vi "Begin.vi"(11 "Image Size":T1=enum."320x240") -> (0 "error out":errorcluster)   [LabVIEW 2012]
doc: "Called before other user functions, this VI is expected to open initial I/O refnums, load in file data, and do all program initialization. Notice that the <B>error out</B> terminal is simply used for data flow. Wiring it to other structures or subVIs ensures that this VI runs first."
uses:
  <vilib>/Rock Robotics/WPI/Camera/WPI_CameraImageSize.ctl
  <vilib>/Rock Robotics/WPI/DriverStation/WPI_DriverStationRobotMode2.ctl
  <vilib>/Rock Robotics/SystemInterfaces/DIO/FPGA_DIOPWMChannel.ctl
  <vilib>/Rock Robotics/WPI/Joystick/WPI_JoystickDeviceEnum.ctl
  <vilib>/Rock Robotics/SystemInterfaces/Typedef/FPGA_TypedefDigitalModule.ctl
  <vilib>/Rock Robotics/WPI/Relay/WPI_RelayDirection.ctl
  <vilib>/Rock Robotics/SystemInterfaces/DIO/FPGA_DIORelayChannel.ctl
  <vilib>/Rock Robotics/SystemInterfaces/AI/FPGA_AIChannel.ctl
  <vilib>/Rock Robotics/SystemInterfaces/AI/FPGA_AIGyroChannel.ctl
  <vilib>/Rock Robotics/SystemInterfaces/DIO/FPGA_DIOChannel.ctl
  <vilib>/Rock Robotics/WPI/Camera/WPI_CameraFrameRate.ctl
  Robot Global Data.vi
  <vilib>/Rock Robotics/WPI/MotorControl/WPI_MotorControlOpen Victor.vi
  <vilib>/Rock Robotics/WPI/Camera/WPI_CameraWhite Balance Values.ctl
  <vilib>/Rock Robotics/WPI/Camera/WPI_CameraExposure Values.ctl
  <vilib>/Rock Robotics/WPI/MotorControl/WPI_MotorControlOpen Jaguar.vi
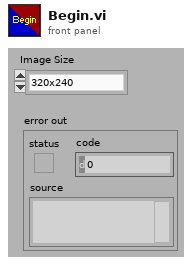
[diagram p1: front panel]
types:
  T1 = typedef "WPI_CameraImageSize.ctl" = enum16{"640x480", "320x240", "160x120"}
  T2 = typedef "FPGA_AIChannel.ctl" = enum8{"AI 1", "AI 2", "AI 3", "AI 4", "AI 5", "AI 6", "AI 7", "AI 8", "Invalid"}
  T3 = typedef "FPGA_DIOChannel.ctl" = enum8{"DIO 1", "DIO 2", "DIO 3", "DIO 4", "DIO 5", "DIO 6", "DIO 7", "DIO 8", "DIO 9", "DIO 10", "DIO 11", "DIO 12", "DIO 13", "DIO 14", "Invalid"}
  T4 = typedef "FPGA_TypedefDigitalModule.ctl" = enum16{"Digital Module 1", "Digital Module 2"}
  T5 = typedef "FPGA_DIOPWMChannel.ctl" = enum8{"PWM 1", "PWM 2", "PWM 3", "PWM 4", "PWM 5", "PWM 6", "PWM 7", "PWM 8", "PWM 9", "PWM 10", "Invalid"}
  T6 = typedef "FPGA_AIGyroChannel.ctl" = enum8{"AI 1", "AI 2", "Invalid"}
  T7 = typedef "FPGA_DIORelayChannel.ctl" = enum8{"Relay 1", "Relay 2", "Relay 3", "Relay 4", "Relay 5", "Relay 6", "Relay 7", "Relay 8", "Invalid"}
  T8 = typedef "WPI_RelayDirection.ctl" = enum16{"Both directions", "Forward only", "Reverse only"}
  T9 = typedef "WPI_JoystickDeviceEnum.ctl" = enum16{"USB 1", "USB 2", "USB 3", "USB 4", "Kinect 1", "Kinect 2"}
  T10 = typedef "WPI_DriverStationRobotMode2.ctl" = enum16{"Autonomous Disabled", "Autonomous Enabled", "Teleop Disabled", "Teleop Enabled", "Timeout", "Finish", "Test Disabled", "Test Enabled"}
  T11 = typedef "WPI_CameraFrameRate.ctl" = u32
  T12 = typedef "WPI_CameraExposure Values.ctl" = enum16{"Auto", "Flicker-free 50 Hz", "Flicker-free 60 Hz", "Hold current"}
  T13 = typedef "WPI_CameraWhite Balance Values.ctl" = enum16{"Auto", "Fixed indoor", "Fixed outdoor 1", "Fixed outdoor 2", "Fixed fluorescent 1", "Fixed fluorescent 2", "Hold current"}
  T14 = typedef "WPI_CameraDevRef.ctl" = cluster{"Camera Address":string, "CameraStatus":errorcluster, "Acquire Image Notifier":refnum<notifier>}
  T15 = typedef "WPI_MotorControlDeviceRef.ctl" = cluster{"DeviceStatus":errorcluster, "Type":enum16{"PWM", "CAN"}, "PWM":cluster{"Digital Module":T4, "PWM Channel":T5, "DeadBand":T16}, "CAN":cluster{"Device Number":u8, "Control Mode":T17, "Semaphore":T18, "Max Vout":dbl}, "Invert":bool, "TransformRef":T19, "InvTransformRef":T19}
  T16 = typedef "WPI_PWMDeadband.ctl" = cluster{"Name":string, "maxPositivePwm":i32, "minPositivePwm":i32, "centerPwm":i32, "maxNegativePwm":i32, "minNegativePwm":i32, "angularRange":u16}
  T17 = typedef "WPI_CANJaguar_ControlMode.ctl" = enum8{"Percent VBus", "Current", "Speed", "Position", "Voltage"}
  T18 = typedef "Semaphore RefNum" = refnum<k1>
  T19 = typedef "WPI_PWMTransform_ConPane.ctl" = refnum<vi>
  T20 = typedef "WPI_JoystickDevRef.ctl" = cluster{"Device":T9}
  T21 = typedef "WPI_ServoDeviceRef.ctl" = cluster{"DeviceStatus":errorcluster, "Digital Module":T4, "PWM Channel":T5, "DeadBand":T16}
  T22 = typedef "WPI_RelayDevRef.ctl" = cluster{"DevStatus":errorcluster, "Relay Channel":T7, "Digital Module":T4, "Relay Direction":T8}
  T23 = typedef "WPI_AnalogChannelDevRef.ctl" = cluster{"DevStatus":errorcluster, "Analog Module":T24, "Analog Channel":T2}
  T24 = typedef "FPGA_TypedefAnalogModule.ctl" = enum16{"Analog Module 1", "Analog Module 2"}
  T25 = typedef "WPI_DigitalInputDevRef.ctl" = cluster{"DevStatus":errorcluster, "DIO Channel":T3, "Digital Module":T4}
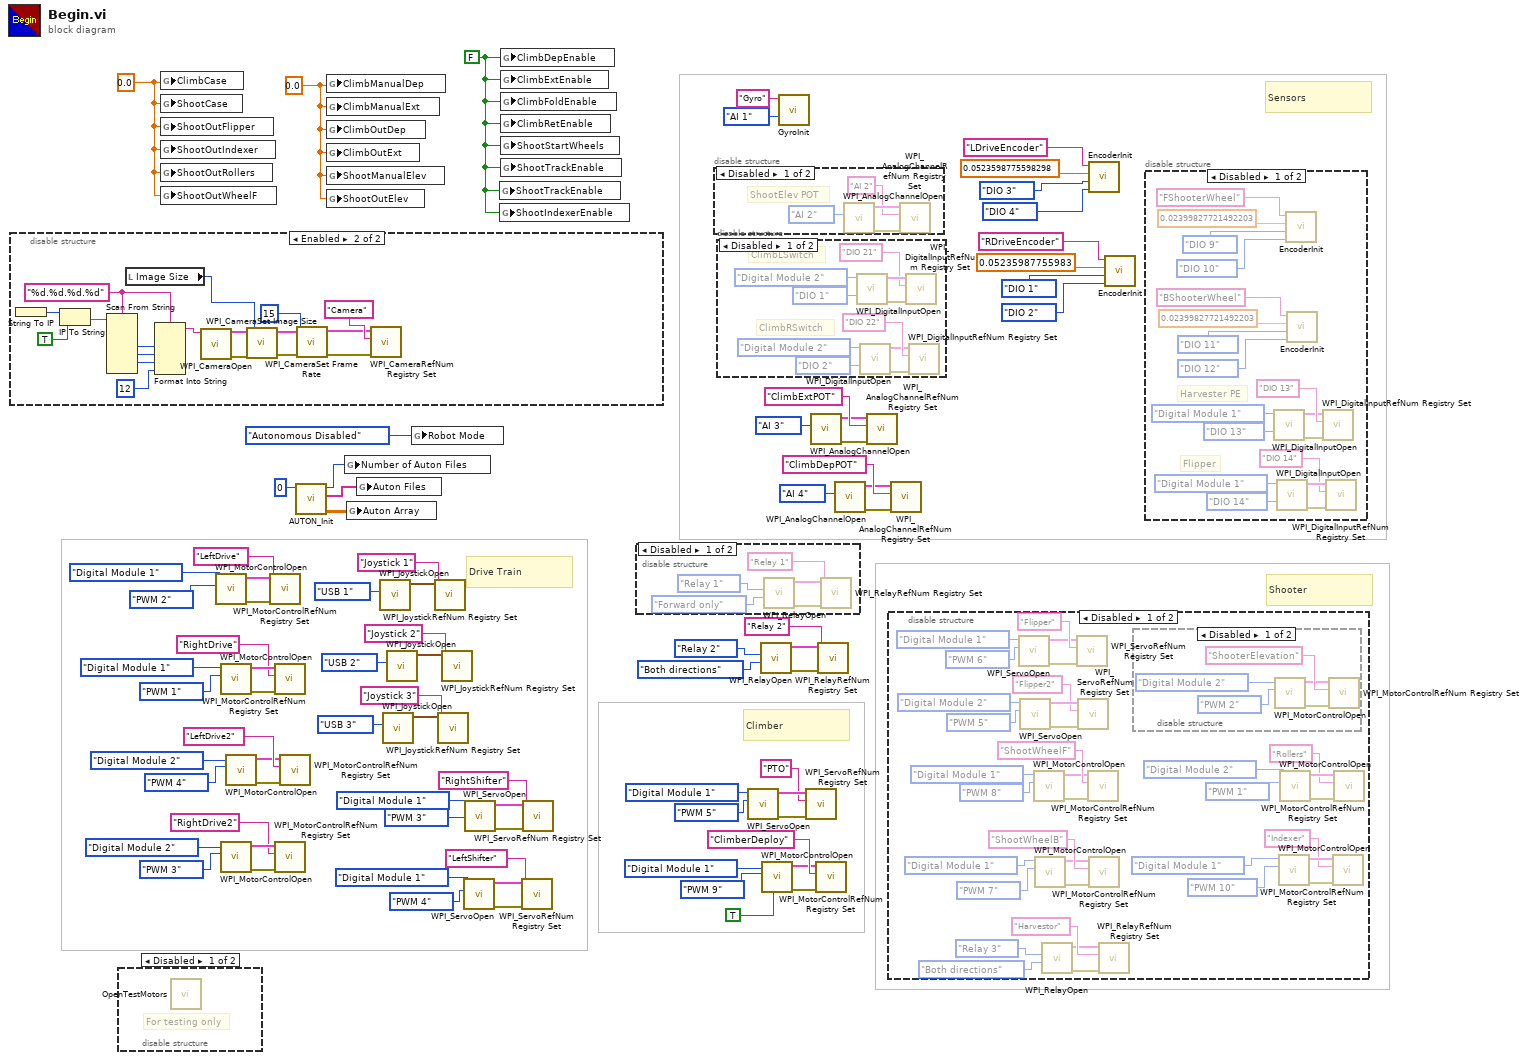
[diagram p0: block diagram]
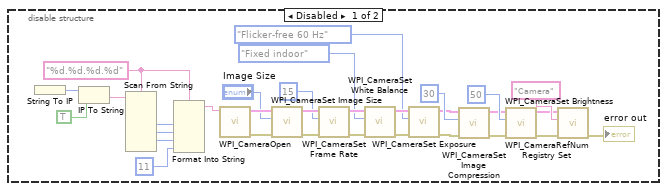
[diagram p6: hidden frame]
diagram:
  w57 = FALSE ("ClimbDepEnable")
  w58 = 0.0 ("ClimbCase")
  w59 = 0.0 ("ClimbCase")
  # "Drive Train"
  # "Climber"
  # "Shooter"
  # "Sensors"
  n1 = disable-structure shown="Enabled" {
    frame Disabled {
      w84 = "%d.%d.%d.%d" ("format string")
      n2 = String To IP() -> (0:w91:u32)  [unwired: 1 in]
      n3 = IP To String(1:TRUE ("dot notation? (F)"), 2:w91) -> (0:w89:string)
      n4 = Scan From String(format string=w84, input string=w89) -> (output 1=w88:i32, output 2=w87:i32, output 3=w86:i32)  [unwired: 7 in, 3 out]
      n5 = Format Into String(format string=w84, w88, w87, w86, 11 ("Compression")) -> (resulting string=w83:string)  [unwired: 2 in, 1 out]
      n6 = call <vilib>:"WPI_CameraOpen.vi"("Camera Address"=w83) -> ("error out"=w103:errorcluster, "CameraDevRef"=w104:T14)  [unwired: 1 in, 8 out]
      n7 = call <vilib>:"WPI_CameraSet Image Size.vi"("error in (no error)"=w103, "Image Size"="Image Size", "CameraDevRef"=w104) -> ("error out"=w102:errorcluster, "CameraDevRef Out"=w105:T14)  [unwired: 7 out]
      n8 = call <vilib>:"WPI_CameraSet Frame Rate.vi"("error in (no error)"=w102, "Frame Rate (fps)"=T11 15, "CameraDevRef"=w105) -> ("error out"=w101:errorcluster, "CameraDevRef Out"=w107:T14)  [unwired: 7 out]
      n9 = call <vilib>:"WPI_CameraSet White Balance.vi"("error in (no error)"=w101, "White Balance"=WPI_CameraWhite_Balance_Values."Fixed indoor", "CameraDevRef"=w107) -> ("error out"=w100:errorcluster, "CameraDevRef Out"=w106:T14)  [unwired: 7 out]
      n10 = call <vilib>:"WPI_CameraSet Exposure.vi"("error in (no error)"=w100, "Exposure"=WPI_CameraExposure_Values."Flicker-free 60 Hz", "CameraDevRef"=w106) -> ("error out"=w99:errorcluster, "CameraDevRef Out"=w109:T14)  [unwired: 7 out]
      n11 = call <vilib>:"WPI_CameraSet Image Compression.vi"("error in (no error)"=w99, "Compression"=30, "CameraDevRef"=w109) -> ("error out"=w98:errorcluster, "CameraDevRef Out"=w108:T14)  [unwired: 7 out]
      n12 = call <vilib>:"WPI_CameraSet Brightness.vi"("error in (no error)"=w98, "Brightness"=50, "CameraDevRef"=w108) -> ("error out"=w96:errorcluster, "CameraDevRef Out"=w97:T14)  [unwired: 7 out]
      n13 = call <vilib>:"WPI_CameraRefNum Registry Set.vi"("error in (no error)"=w96, "refnum name"="Camera", "CameraDevRef"=w97) -> ("error out"=→"error out":errorcluster)  [unwired: 8 out]
    }
    frame Enabled {
      w122 = "%d.%d.%d.%d" ("format string")
      n14 = String To IP() -> (0:w129:u32)  [unwired: 1 in]
      n15 = IP To String(1:TRUE ("dot notation? (F)"), 2:w129) -> (0:w127:string)
      n16 = Scan From String(format string=w122, input string=w127) -> (output 1=w126:i32, output 2=w125:i32, output 3=w124:i32)  [unwired: 7 in, 3 out]
      n17 = local read "Image Size"() -> (w118:T1)
      n18 = Format Into String(format string=w122, w126, w125, w124, 12 ("Compression")) -> (resulting string=w121:string)  [unwired: 2 in, 1 out]
      n19 = call <vilib>:"WPI_CameraOpen.vi"("Camera Address"=w121) -> ("error out"=w120:errorcluster, "CameraDevRef"=w119:T14)  [unwired: 1 in, 8 out]
      n20 = call <vilib>:"WPI_CameraSet Image Size.vi"("error in (no error)"=w120, "Image Size"=w118, "CameraDevRef"=w119) -> ("error out"=w116:errorcluster, "CameraDevRef Out"=w117:T14)  [unwired: 7 out]
      n21 = call <vilib>:"WPI_CameraSet Frame Rate.vi"("error in (no error)"=w116, "Frame Rate (fps)"=T11 15, "CameraDevRef"=w117) -> ("error out"=w115:errorcluster, "CameraDevRef Out"=w114:T14)  [unwired: 7 out]
      n22 = call <vilib>:"WPI_CameraRefNum Registry Set.vi"("error in (no error)"=w115, "refnum name"="Camera", "CameraDevRef"=w114) -> ()  [unwired: 9 out]
    }
  }
  n23 = disable-structure shown="Disabled" {
    frame Disabled {
      # "For testing only"
      n24 = call "OpenTestMotors.vi"() -> ()  [unwired: 12 in]
    }
    frame Enabled {
    }
  }
  n25 = global write "Robot Global Data.vi" "ClimbCase"(w59) -> ()
  n26 = global write "Robot Global Data.vi" "ShootCase"(w59) -> ()
  n27 = global write "Robot Global Data.vi" "ShootOutFlipper"(w59) -> ()
  n28 = global write "Robot Global Data.vi" "ShootOutIndexer"(w59) -> ()
  n29 = global write "Robot Global Data.vi" "ShootOutRollers"(w59) -> ()
  n30 = global write "Robot Global Data.vi" "ShootOutWheelF"(w59) -> ()
  n31 = call-poly <vilib>:"WPI_MotorControlOpen.vi"("PWM Channel"=FPGA_DIOPWMChannel."PWM 2", "Digital Module (Module 1)"=FPGA_TypedefDigitalModule."Digital Module 1") -> ("error out"=w69:errorcluster, "MotorControlDeviceRef"=w70:T15)  [unwired: 8 in]
  n32 = call-poly <vilib>:"WPI_MotorControlOpen.vi"("PWM Channel"=FPGA_DIOPWMChannel."PWM 1", "Digital Module (Module 1)"=FPGA_TypedefDigitalModule."Digital Module 1") -> ("error out"=w76:errorcluster, "MotorControlDeviceRef"=w75:T15)  [unwired: 8 in]
  n33 = call-poly <vilib>:"WPI_MotorControlOpen.vi"("PWM Channel"=FPGA_DIOPWMChannel."PWM 3", "Digital Module (Module 1)"=FPGA_TypedefDigitalModule."Digital Module 2") -> ("error out"=w55:errorcluster, "MotorControlDeviceRef"=w54:T15)  [unwired: 8 in]
  n34 = call-poly <vilib>:"WPI_MotorControlOpen.vi"("PWM Channel"=FPGA_DIOPWMChannel."PWM 4", "Digital Module (Module 1)"=FPGA_TypedefDigitalModule."Digital Module 2") -> ("error out"=w46:errorcluster, "MotorControlDeviceRef"=w47:T15)  [unwired: 8 in]
  n35 = call <vilib>:"WPI_MotorControlRefNum Registry Set.vi"("error in (no error)"=w69, "refnum name"="LeftDrive", "MotorControlDevRef"=w70) -> ()  [unwired: 7 in, 2 out]
  n36 = call <vilib>:"WPI_MotorControlRefNum Registry Set.vi"("error in (no error)"=w76, "refnum name"="RightDrive", "MotorControlDevRef"=w75) -> ()  [unwired: 7 in, 2 out]
  n37 = call <vilib>:"WPI_MotorControlRefNum Registry Set.vi"("error in (no error)"=w55, "refnum name"="RightDrive2", "MotorControlDevRef"=w54) -> ()  [unwired: 7 in, 2 out]
  n38 = call <vilib>:"WPI_MotorControlRefNum Registry Set.vi"("error in (no error)"=w46, "refnum name"="LeftDrive2", "MotorControlDevRef"=w47) -> ()  [unwired: 7 in, 2 out]
  n39 = call "AUTON_Init.vi"("Default File"=0) -> ("Auton Array"=w77:dbl[][], "Auton Files"=w78:string[], "Number of Auton Files"=w79:i64)  [unwired: 8 in]
  n40 = global write "Robot Global Data.vi" "ClimbManualDep"(w58) -> ()
  n41 = global write "Robot Global Data.vi" "ClimbManualExt"(w58) -> ()
  n42 = global write "Robot Global Data.vi" "ClimbOutDep"(w58) -> ()
  n43 = global write "Robot Global Data.vi" "ClimbOutExt"(w58) -> ()
  n44 = global write "Robot Global Data.vi" "ShootManualElev"(w58) -> ()
  n45 = global write "Robot Global Data.vi" "ShootOutElev"(w58) -> ()
  n46 = global write "Robot Global Data.vi" "Number of Auton Files"(w79) -> ()
  n47 = global write "Robot Global Data.vi" "Auton Array"(w77) -> ()
  n48 = global write "Robot Global Data.vi" "Auton Files"(w78) -> ()
  n49 = call <vilib>:"WPI_JoystickOpen.vi"("JoystickDevice"=WPI_JoystickDeviceEnum."USB 1") -> ("JoystickDevRef"=w60:T20)  [unwired: 10 in]
  n50 = call <vilib>:"WPI_JoystickOpen.vi"("JoystickDevice"=WPI_JoystickDeviceEnum."USB 3") -> ("JoystickDevRef"=w66:T20)  [unwired: 10 in]
  n51 = call <vilib>:"WPI_JoystickOpen.vi"("JoystickDevice"=WPI_JoystickDeviceEnum."USB 2") -> ("JoystickDevRef"=w65:T20)  [unwired: 10 in]
  n52 = global write "Robot Global Data.vi" "Robot Mode"(WPI_DriverStationRobotMode2."Autonomous Disabled" ("Robot Mode")) -> ()
  n53 = call <vilib>:"WPI_JoystickRefNum Registry Set.vi"("refnum name"="Joystick 1", "JoystickDevRef"=w60) -> ()  [unwired: 8 in, 2 out]
  n54 = call <vilib>:"WPI_JoystickRefNum Registry Set.vi"("refnum name"="Joystick 3", "JoystickDevRef"=w66) -> ()  [unwired: 8 in, 2 out]
  n55 = call <vilib>:"WPI_JoystickRefNum Registry Set.vi"("refnum name"="Joystick 2", "JoystickDevRef"=w65) -> ()  [unwired: 8 in, 2 out]
  n56 = call <vilib>:"WPI_ServoOpen.vi"("PWM Channel"=FPGA_DIOPWMChannel."PWM 4", "Digital Module (Module 1)"=FPGA_TypedefDigitalModule."Digital Module 1") -> ("error out"=w39:errorcluster, "ServoDeviceRef"=w32:T21)  [unwired: 8 in]
  n57 = call <vilib>:"WPI_ServoOpen.vi"("PWM Channel"=FPGA_DIOPWMChannel."PWM 3", "Digital Module (Module 1)"=FPGA_TypedefDigitalModule."Digital Module 1") -> ("error out"=w38:errorcluster, "ServoDeviceRef"=w37:T21)  [unwired: 8 in]
  n58 = global write "Robot Global Data.vi" "ShootTrackEnable"(w57) -> ()
  n59 = global write "Robot Global Data.vi" "ShootIndexerEnable"(w57) -> ()
  n60 = global write "Robot Global Data.vi" "ClimbDepEnable"(w57) -> ()
  n61 = global write "Robot Global Data.vi" "ClimbExtEnable"(w57) -> ()
  n62 = global write "Robot Global Data.vi" "ClimbFoldEnable"(w57) -> ()
  n63 = global write "Robot Global Data.vi" "ClimbRetEnable"(w57) -> ()
  n64 = global write "Robot Global Data.vi" "ShootStartWheels"(w57) -> ()
  n65 = global write "Robot Global Data.vi" "ShootTrackEnable"(w57) -> ()
  n66 = call <vilib>:"WPI_ServoRefNum Registry Set.vi"("error in (no error)"=w39, "refnum name"="LeftShifter", "ServoDeviceRef"=w32) -> ()  [unwired: 7 in, 2 out]
  n67 = call <vilib>:"WPI_ServoRefNum Registry Set.vi"("error in (no error)"=w38, "refnum name"="RightShifter", "ServoDeviceRef"=w37) -> ()  [unwired: 7 in, 2 out]
  n68 = disable-structure shown="Disabled" {
    frame Disabled {
      n69 = call <vilib>:"WPI_RelayOpen.vi"("Relay Direction"=WPI_RelayDirection."Forward only", "Relay Channel"=FPGA_DIORelayChannel."Relay 1") -> ("error out"=w135:errorcluster, "RelayDevRef"=w134:T22)  [unwired: 8 in]
      n70 = call <vilib>:"WPI_RelayRefNum Registry Set.vi"("error in (no error)"=w135, "refnum name"="Relay 1", "RelayDevRef"=w134) -> ()  [unwired: 7 in, 2 out]
    }
    frame Enabled {
    }
  }
  n71 = disable-structure shown="Disabled" {
    frame Disabled {
      # "ShootElev POT"
      n72 = call <vilib>:"WPI_AnalogChannelOpen.vi"("Analog Channel"=FPGA_AIChannel."AI 2") -> ("error out"=w136:errorcluster, "AIDeviceRef"=w138:T23)  [unwired: 9 in]
      n73 = call <vilib>:"WPI_AnalogChannelRefNum Registry Set.vi"("error in (no error)"=w136, "refnum name"="AI 2", "AIDeviceRef"=w138) -> ()  [unwired: 7 in, 2 out]
    }
    frame Enabled {
    }
  }
  n74 = disable-structure shown="Disabled" {
    frame Disabled {
      # "ClimbRSwitch"
      # "ClimbLSwitch"
      n75 = call <vilib>:"WPI_DigitalInputOpen.vi"("DIO Channel"=FPGA_DIOChannel."DIO 1", "Digital Module (Module 1)"=FPGA_TypedefDigitalModule."Digital Module 2") -> ("error out"=w141:errorcluster, "DigitalInputDevRef"=w142:T25)  [unwired: 8 in]
      n76 = call <vilib>:"WPI_DigitalInputOpen.vi"("DIO Channel"=FPGA_DIOChannel."DIO 2", "Digital Module (Module 1)"=FPGA_TypedefDigitalModule."Digital Module 2") -> ("error out"=w148:errorcluster, "DigitalInputDevRef"=w147:T25)  [unwired: 8 in]
      n77 = call <vilib>:"WPI_DigitalInputRefNum Registry Set.vi"("error in (no error)"=w141, "refnum name"="DIO 21", "DigitalInputDevRef"=w142) -> ()  [unwired: 7 in, 2 out]
      n78 = call <vilib>:"WPI_DigitalInputRefNum Registry Set.vi"("error in (no error)"=w148, "refnum name"="DIO 22", "DigitalInputDevRef"=w147) -> ()  [unwired: 7 in, 2 out]
    }
    frame Enabled {
    }
  }
  n79 = call <vilib>:"WPI_ServoOpen.vi"("PWM Channel"=FPGA_DIOPWMChannel."PWM 5", "Digital Module (Module 1)"=FPGA_TypedefDigitalModule."Digital Module 1") -> ("error out"=w17:errorcluster, "ServoDeviceRef"=w16:T21)  [unwired: 8 in]
  n80 = call <vilib>:"WPI_RelayOpen.vi"("Relay Direction"=WPI_RelayDirection."Both directions", "Relay Channel"=FPGA_DIORelayChannel."Relay 2") -> ("error out"=w40:errorcluster, "RelayDevRef"=w41:T22)  [unwired: 8 in]
  n81 = call-poly <vilib>:"WPI_MotorControlOpen.vi"("Invert"=TRUE, "PWM Channel"=FPGA_DIOPWMChannel."PWM 9", "Digital Module (Module 1)"=FPGA_TypedefDigitalModule."Digital Module 1") -> ("error out"=w22:errorcluster, "MotorControlDeviceRef"=w21:T15)  [unwired: 7 in]
  n82 = call "GyroInit.vi"("refnum name"="Gyro", "Analog Channel"=FPGA_AIGyroChannel."AI 1") -> ()  [unwired: 8 in]
  n83 = call <vilib>:"WPI_ServoRefNum Registry Set.vi"("error in (no error)"=w17, "refnum name"="PTO", "ServoDeviceRef"=w16) -> ()  [unwired: 7 in, 2 out]
  n84 = call <vilib>:"WPI_AnalogChannelOpen.vi"("Analog Channel"=FPGA_AIChannel."AI 3") -> ("error out"=w1:errorcluster, "AIDeviceRef"=w2:T23)  [unwired: 9 in]
  n85 = call <vilib>:"WPI_MotorControlRefNum Registry Set.vi"("error in (no error)"=w22, "refnum name"="ClimberDeploy", "MotorControlDevRef"=w21) -> ()  [unwired: 7 in, 2 out]
  n86 = call <vilib>:"WPI_RelayRefNum Registry Set.vi"("error in (no error)"=w40, "refnum name"="Relay 2", "RelayDevRef"=w41) -> ()  [unwired: 7 in, 2 out]
  n87 = call <vilib>:"WPI_AnalogChannelOpen.vi"("Analog Channel"=FPGA_AIChannel."AI 4") -> ("error out"=w26:errorcluster, "AIDeviceRef"=w27:T23)  [unwired: 9 in]
  n88 = call <vilib>:"WPI_AnalogChannelRefNum Registry Set.vi"("error in (no error)"=w1, "refnum name"="ClimbExtPOT", "AIDeviceRef"=w2) -> ()  [unwired: 7 in, 2 out]
  n89 = disable-structure shown="Disabled" {
    frame Disabled {
      n90 = call <vilib>:"WPI_ServoOpen.vi"("PWM Channel"=FPGA_DIOPWMChannel."PWM 6", "Digital Module (Module 1)"=FPGA_TypedefDigitalModule."Digital Module 1") -> ("error out"=w170:errorcluster, "ServoDeviceRef"=w171:T21)  [unwired: 8 in]
      n91 = call <vilib>:"WPI_ServoOpen.vi"("PWM Channel"=FPGA_DIOPWMChannel."PWM 5", "Digital Module (Module 1)"=FPGA_TypedefDigitalModule."Digital Module 2") -> ("error out"=w169:errorcluster, "ServoDeviceRef"=w168:T21)  [unwired: 8 in]
      n92 = call-poly <vilib>:"WPI_MotorControlOpen.vi"("PWM Channel"=FPGA_DIOPWMChannel."PWM 8", "Digital Module (Module 1)"=FPGA_TypedefDigitalModule."Digital Module 1") -> ("error out"=w156:errorcluster, "MotorControlDeviceRef"=w157:T15)  [unwired: 8 in]
      n93 = call-poly <vilib>:"WPI_MotorControlOpen.vi"("PWM Channel"=FPGA_DIOPWMChannel."PWM 7", "Digital Module (Module 1)"=FPGA_TypedefDigitalModule."Digital Module 1") -> ("error out"=w152:errorcluster, "MotorControlDeviceRef"=w151:T15)  [unwired: 8 in]
      n94 = call <vilib>:"WPI_RelayOpen.vi"("Relay Direction"=WPI_RelayDirection."Both directions", "Relay Channel"=FPGA_DIORelayChannel."Relay 3") -> ("error out"=w160:errorcluster, "RelayDevRef"=w161:T22)  [unwired: 8 in]
      n95 = call <vilib>:"WPI_ServoRefNum Registry Set.vi"("error in (no error)"=w170, "refnum name"="Flipper", "ServoDeviceRef"=w171) -> ()  [unwired: 7 in, 2 out]
      n96 = call <vilib>:"WPI_ServoRefNum Registry Set.vi"("error in (no error)"=w169, "refnum name"="Flipper2", "ServoDeviceRef"=w168) -> ()  [unwired: 7 in, 2 out]
      n97 = call <vilib>:"WPI_MotorControlRefNum Registry Set.vi"("error in (no error)"=w156, "refnum name"="ShootWheelF", "MotorControlDevRef"=w157) -> ()  [unwired: 7 in, 2 out]
      n98 = call <vilib>:"WPI_MotorControlRefNum Registry Set.vi"("error in (no error)"=w152, "refnum name"="ShootWheelB", "MotorControlDevRef"=w151) -> ()  [unwired: 7 in, 2 out]
      n99 = call <vilib>:"WPI_RelayRefNum Registry Set.vi"("error in (no error)"=w160, "refnum name"="Harvestor", "RelayDevRef"=w161) -> ()  [unwired: 7 in, 2 out]
      n100 = disable-structure shown="Disabled" {
        frame Disabled {
          n101 = call-poly <vilib>:"WPI_MotorControlOpen.vi"("PWM Channel"=FPGA_DIOPWMChannel."PWM 2", "Digital Module (Module 1)"=FPGA_TypedefDigitalModule."Digital Module 2") -> ("error out"=w187:errorcluster, "MotorControlDeviceRef"=w186:T15)  [unwired: 8 in]
          n102 = call <vilib>:"WPI_MotorControlRefNum Registry Set.vi"("error in (no error)"=w187, "refnum name"="ShooterElevation", "MotorControlDevRef"=w186) -> ()  [unwired: 7 in, 2 out]
        }
        frame Enabled {
        }
      }
      n103 = call-poly <vilib>:"WPI_MotorControlOpen.vi"("PWM Channel"=FPGA_DIOPWMChannel."PWM 10", "Digital Module (Module 1)"=FPGA_TypedefDigitalModule."Digital Module 1") -> ("error out"=w177:errorcluster, "MotorControlDeviceRef"=w178:T15)  [unwired: 8 in]
      n104 = call-poly <vilib>:"WPI_MotorControlOpen.vi"("PWM Channel"=FPGA_DIOPWMChannel."PWM 1", "Digital Module (Module 1)"=FPGA_TypedefDigitalModule."Digital Module 2") -> ("error out"=w182:errorcluster, "MotorControlDeviceRef"=w183:T15)  [unwired: 8 in]
      n105 = call <vilib>:"WPI_MotorControlRefNum Registry Set.vi"("error in (no error)"=w177, "refnum name"="Indexer", "MotorControlDevRef"=w178) -> ()  [unwired: 7 in, 2 out]
      n106 = call <vilib>:"WPI_MotorControlRefNum Registry Set.vi"("error in (no error)"=w182, "refnum name"="Rollers", "MotorControlDevRef"=w183) -> ()  [unwired: 7 in, 2 out]
    }
    frame Enabled {
    }
  }
  n107 = call <vilib>:"WPI_AnalogChannelRefNum Registry Set.vi"("error in (no error)"=w26, "refnum name"="ClimbDepPOT", "AIDeviceRef"=w27) -> ()  [unwired: 7 in, 2 out]
  n108 = call "EncoderInit.vi"("refnum name"="LDriveEncoder", "DistancePerCount"=0.0523598775598298, "DIO Channel"=FPGA_DIOChannel."DIO 3", "DIO Channel 2"=FPGA_DIOChannel."DIO 4") -> ()  [unwired: 7 in]
  n109 = call "EncoderInit.vi"("refnum name"="RDriveEncoder", "DistancePerCount"=0.05235987755983, "DIO Channel"=FPGA_DIOChannel."DIO 1", "DIO Channel 2"=FPGA_DIOChannel."DIO 2") -> ()  [unwired: 7 in]
  n110 = disable-structure shown="Disabled" {
    frame Disabled {
      # "Flipper"
      # "Harvester PE"
      n111 = call <vilib>:"WPI_DigitalInputOpen.vi"("DIO Channel"=FPGA_DIOChannel."DIO 13", "Digital Module (Module 1)"=FPGA_TypedefDigitalModule."Digital Module 1") -> ("error out"=w198:errorcluster, "DigitalInputDevRef"=w197:T25)  [unwired: 8 in]
      n112 = call <vilib>:"WPI_DigitalInputOpen.vi"("DIO Channel"=FPGA_DIOChannel."DIO 14", "Digital Module (Module 1)"=FPGA_TypedefDigitalModule."Digital Module 1") -> ("error out"=w191:errorcluster, "DigitalInputDevRef"=w192:T25)  [unwired: 8 in]
      n113 = call "EncoderInit.vi"("refnum name"="FShooterWheel", "DistancePerCount"=0.02399827721492203, "DIO Channel"=FPGA_DIOChannel."DIO 9", "DIO Channel 2"=FPGA_DIOChannel."DIO 10") -> ()  [unwired: 7 in]
      n114 = call "EncoderInit.vi"("refnum name"="BShooterWheel", "DistancePerCount"=0.02399827721492203, "DIO Channel"=FPGA_DIOChannel."DIO 11", "DIO Channel 2"=FPGA_DIOChannel."DIO 12") -> ()  [unwired: 7 in]
      n115 = call <vilib>:"WPI_DigitalInputRefNum Registry Set.vi"("error in (no error)"=w198, "refnum name"="DIO 13", "DigitalInputDevRef"=w197) -> ()  [unwired: 7 in, 2 out]
      n116 = call <vilib>:"WPI_DigitalInputRefNum Registry Set.vi"("error in (no error)"=w191, "refnum name"="DIO 14", "DigitalInputDevRef"=w192) -> ()  [unwired: 7 in, 2 out]
    }
    frame Enabled {
    }
  }
